vi "FRCts20_WebMethods_Team_DELETE.vi"(7 "httpRequestID":u32, 11 "team":string) -> ()   [LabVIEW 2014, in "FRCts20_WebMethods.lvlib"]
doc: "<B>DELETE</B> the specified <B>team</B> resource\n\nhttp://<server address>:<port>/FRCts/team/<B>team</B>\n\n{requires authentication}"
uses:
  FRCts20_WebMethods.lvlib
  Backend/source/VI Source/FRCts20_Backend_API/FRCts20_Backend_API_Team.ctl
  Backend/source/VI Source/FRCts20_Backend_API/FRCts20_Backend_API_SW.ctl
  Backend/source/VI Source/FRCts20_Backend_API/FRCts20_Backend_API_Status.ctl
  Backend/source/VI Source/FRCts20_Backend_API/FRCts20_Backend_API_Command_Team.ctl
  Backend/source/VI Source/FRCts20_Backend_API/FRCts20_Backend_API_Team.vi
  <vilib>/wsapi/NI_WebServices.lvlib
  Backend/source/VI Source/FRCts20_Backend_API/FRCts20_Backend_API.lvlib
panel:
  in  "query":string
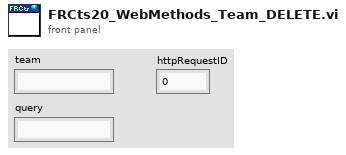
[diagram p1: front panel]
types:
  T1 = typedef "FRCts20_Backend_API.lvlib/FRCts20_Backend_API_Command_Team.ctl" = string
  T2 = typedef "FRCts20_Backend_API.lvlib/FRCts20_Backend_API_Team.ctl" = cluster{"Team Index":u32, "Team Number":u32, "Team Name":string, "Short Team Name":string, "Nick Name":string, "Robot Name":string, "City":string, "State":string, "Country":string, "Rookie Year":u32, "SWType":T3, "CAN":bool, "Vision":bool, "Kinect":bool, "Tags":string, "Avatar":string, "Request Array":cluster{"Request Index":u32, "Description":string, "Status":T4, "Open Date":timestamp, "Last Update":timestamp, "Close Date":timestamp}[], "Events Attending":cluster{"EventIndex":dbl, "EventName":string, "IsLive":bool}[], "APIReturn":string}
  T3 = typedef "FRCts20_Backend_API.lvlib/FRCts20_Backend_API_SW.ctl" = string
  T4 = typedef "FRCts20_Backend_API.lvlib/FRCts20_Backend_API_Status.ctl" = enum16{"Open", "In Work", "Closed"}
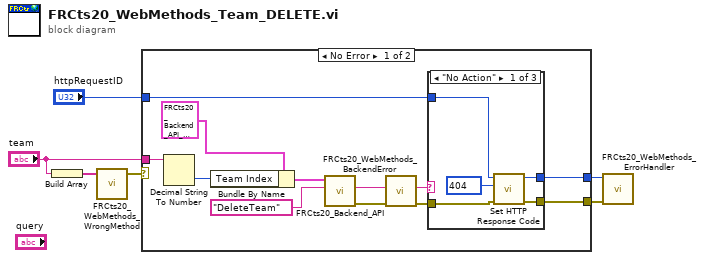
[diagram p0: block diagram]
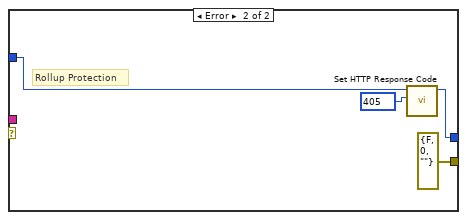
[diagram p4: hidden frame]
diagram:
  n1 = Build Array("team") -> (w2:string[])
  n2 = call "FRCts20_WebMethods_WrongMethod.vi"("Method Inputs"=w2) -> ("error out"=w1:errorcluster)  [unwired: 4 in]
  n3 = case shown="No Error" w1 {
    tunnel: "httpRequestID" -> [w8 w31]
    tunnel: "team" -> [w18 _]
    tunnel: [w9 errorcluster {"status"=FALSE, "code"=0, "source"=""} ("error out")] -> w4
    tunnel: [w7 w29] -> w3
    frame No Error {
      n4 = Decimal String To Number(string=w18) -> (number=w16:i32)  [unwired: 2 in, 1 out]
      n5 = Bundle By Name(cluster=T2 {"Team Index"=0, "Team Number"=0, "Team Name"="", "Short Team Name"="", "Nick Name"="", "Robot Name"="", "City"="", "State"="", "Country"="", "Rookie Year"=0, "SWType"="", "CAN"=FALSE, "Vision"=FALSE, "Kinect"=FALSE, "Tags"="", "Avatar"="", "Request Array"=[], "Events Attending"=[], "APIReturn"=""} ("Team"), "Team Index"=w16) -> (w15:T2)
      n6 = call-poly "FRCts20_Backend_API.vi"("Command"=T1 "DeleteTeam", "Team In"=w15) -> ("error out"=w13:errorcluster, "Status"=w12:string)  [unwired: 7 in, 1 out]
      n7 = call "FRCts20_WebMethods_BackendError.vi"("error in (no error)"=w13, "Status"=w12) -> ("error out"=w10:errorcluster, "Status out"=w11:string)  [unwired: 8 in]
      n8 = case shown="\"No Action\"" w11 {
        tunnel: w10 -> [w20 w25 w27]
        tunnel: [w23 w25 w27] -> w9
        tunnel: w8 -> [w21 w24 w26]
        tunnel: [w22 w24 w26] -> w7
        frame "No Action" {
          w19 = 404 items=["100"=100, "101"=101, "200"=200, "201"=201, "202"=202, "203"=203, "204"=204, "205"=205, "206"=206, "300"=300, "301"=301, "302"=302, "303"=303, "304"=304, "305"=305, "306"=306, "307"=307, "400"=400, "401"=401, "402"=402, "403"=403, "404"=404, "405"=405, "406"=406, "407"=407, "408"=408, "409"=409, "410"=410, "411"=411, "412"=412, "413"=413, "414"=414, "415"=415, "416"=416, "417"=417, "500"=500, "501"=501, "502"=502, "503"=503, "504"=504, "505"=505] ("response code (200)")
          n9 = call <vilib>:"Set HTTP Response Code.vi"("error in (no error)"=w20, "response code (200)"=w19, "httpRequestID"=w21) -> ("error out"=w23:errorcluster, "httpRequestID out"=w22:u32)  [unwired: 7 in]
        }
        frame "Backend Error", Default {
        }
        frame "Success" {
        }
      }
    }
    frame Error {
      w30 = 405 items=["100"=100, "101"=101, "200"=200, "201"=201, "202"=202, "203"=203, "204"=204, "205"=205, "206"=206, "300"=300, "301"=301, "302"=302, "303"=303, "304"=304, "305"=305, "306"=306, "307"=307, "400"=400, "401"=401, "402"=402, "403"=403, "404"=404, "405"=405, "406"=406, "407"=407, "408"=408, "409"=409, "410"=410, "411"=411, "412"=412, "413"=413, "414"=414, "415"=415, "416"=416, "417"=417, "500"=500, "501"=501, "502"=502, "503"=503, "504"=504, "505"=505] ("response code (200)")
      # "Rollup Protection"
      n10 = call <vilib>:"Set HTTP Response Code.vi"("response code (200)"=w30, "httpRequestID"=w31) -> ("httpRequestID out"=w29:u32)  [unwired: 8 in, 1 out]
    }
  }
  n11 = call "FRCts20_WebMethods_ErrorHandler.vi"("error in"=w4, "httpRequestID"=w3) -> ()  [unwired: 9 in, 1 out]
